vi "Global.vi"() -> ()   [LabVIEW 2017, in "GE_RM_Shared.lvlib"]
uses:
  RefMem DMA Configuration.llb/GE_RM_Shared.lvlib
panel:
  out "CSV File Path":string="CSV File Path"
  in  "Compiled.Settings":string="Compiled.Settings"
  out "Decimation Channel GUID":string="8433dcab-dea3-4110-97cf-311a1b3fd76d"
  out "Block Address":string="Block Address"
  out "CPU":string="CPU"
  out "Type":string="Type"
  out "Main Page GUID":string="1d8f030b-140c-49c3-a487-fe6eca8ef735"
  out "Status Section GUID":string="782d9ef4-3de5-4e4c-bb43-83b54ca0e2a2"
  out "VISA Name":string="VISA Name"
  out "Relative Address in Block":string="Relative Address in Block"
  out "Del Prot Chan GUID":string="e91a84f3-78c7-400a-8e17-8c81a2c16c94"
  out "Data Channel GUID":string="44f71a1c-f40f-4d80-99bc-9ce0de59748b"
  out "Data Folder GUID":string="46fff8b9-14f1-4a93-83c9-fa3107fe490e"
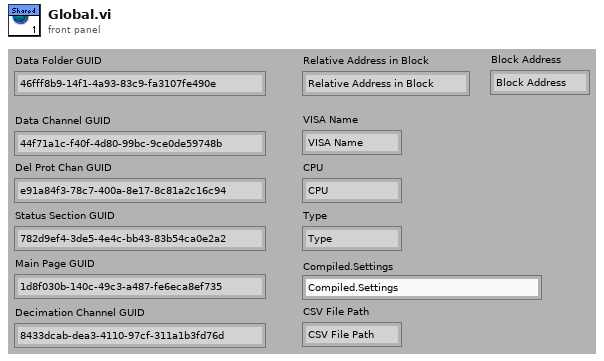
[diagram p1: front panel]
diagram:
